vi "Task Init.vi"(8 "error in (no error)":errorcluster, 11 "DaqDigitalIn in":refnum<class "DaqDigitalIn.lvclass">) -> (0 "error out":errorcluster, 3 "DaqDigitalIn out":refnum<class "DaqDigitalIn.lvclass">)   [LabVIEW 2020, in "VolatusDaq.lvlib" / "DaqDigitalIn.lvclass"]
uses:
  DaqDigitalIn.lvclass
  DaqDigitalIn.lvclass/DaqDigitalIn.ctl
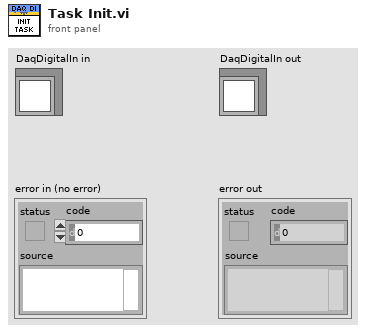
[diagram p1: front panel]
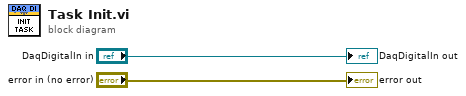
[diagram p0: block diagram]
diagram:
  "error out" <- "error in (no error)"
  "DaqDigitalIn out" <- "DaqDigitalIn in"
